vi "JSON to LVObject.vi"(7 "Flatten To JSON Object in":refnum<class "Flatten To JSON Object.lvclass">, 8 "error in (no error)":errorcluster, 9 "Object Type":refnum<class>, 10 "Offset":i32, 11 "JSON":string) -> (0 "error out":errorcluster, 1 "Object":refnum<class>)   [LabVIEW 2017, in "Flatten To JSON Object.lvclass"]
uses:
  Flatten To JSON Object.lvclass
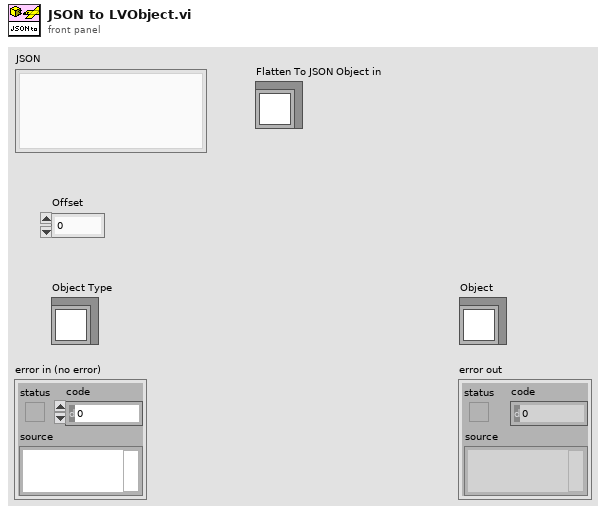
[diagram p1: front panel]
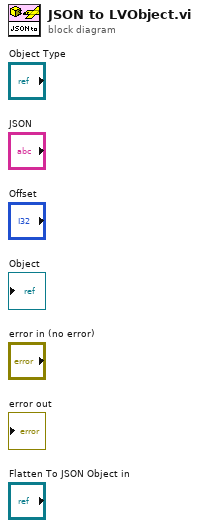
[diagram p0: block diagram]
diagram:
